vi "potential field obstacle avoidence.vi"(8 "F constant":i16, 11 "LIDAR raw data":u8) -> (3 "scan complete?":bool)   [LabVIEW 2010]
panel:
  in  "vehicle Fx":fxp<+/-,16,13> format="%.7g"
  in  "vehicle Fy":fxp<+/-,16,13> format="%.7g"
  out "F angle":i8
  out "F magnitude":i16
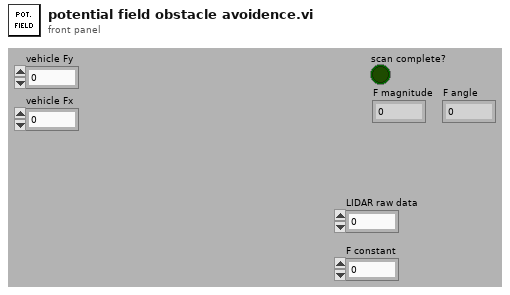
[diagram p1: front panel]
types:
  T1 = enum16{"confirm check sum", "check status byte", "read measured values", "confirm measurement", "confirm command", "read message length", "read address", "wait for \"02\""}
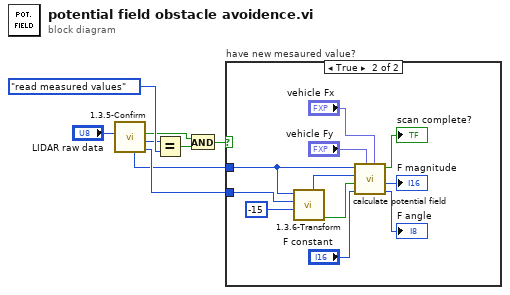
[diagram p0: block diagram]
diagram:
  n1 = call "1.3.5-Confirm.vi"("LIDAR raw data"="LIDAR raw data") -> ("last measured value"=w3:u16, "parser state"=w5:T1, "new value?"=w6:bool, "angle"=w2:u8)  [unwired: 7 in]
  n2 = Equal?(x=w5, y=T1."read measured values" ("parser state")) -> (x = y?=w8:bool)
  n3 = And(x=w6, y=w8) -> (x .and. y?=w4:bool)
  n4 = case "have new mesaured value?" shown="True" w4 {
    tunnel: w3 -> [_ w19]
    tunnel: w2 -> [_ w17]
    frame False {
    }
    frame True {
      n5 = call "1.3.6-Transform.vi"("Lidar Vertical Position"=i8 -15, "Lidar Distance"=w19, "Lidar Scan Angle"=w17) -> ("Is object?"=w15:bool, "object distance squared"=w16:i16)  [unwired: 3 in, 4 out]
      n6 = call "calculate potential field.vi"("vehicle Fx"="vehicle Fx", "vehicle Fy"="vehicle Fy", "F constant"="F constant", "Is object?"=w15, "object distance squared"=w16, "angle"=w17) -> ("F angle"=→"F angle":i8, "F magnitude"=→"F magnitude":i16, "scan complete?"=→"scan complete?":bool)  [unwired: 3 in]
    }
  }
